vi "Untitled 6сщзн.vi"() -> ()   [LabVIEW 2021]
panel:
  in  "На улице":dbl
  in  "stop":bool
  out "XY Graph":cluster{i32[], dbl[]}[](graph)
  in  "Установка":dbl
  out "I":dbl
  in  "dt":dbl
  out "Даткчик":dbl
  out "IprevErr":dbl
  in  "kp":dbl
  in  "ki":dbl
  in  "kd":dbl
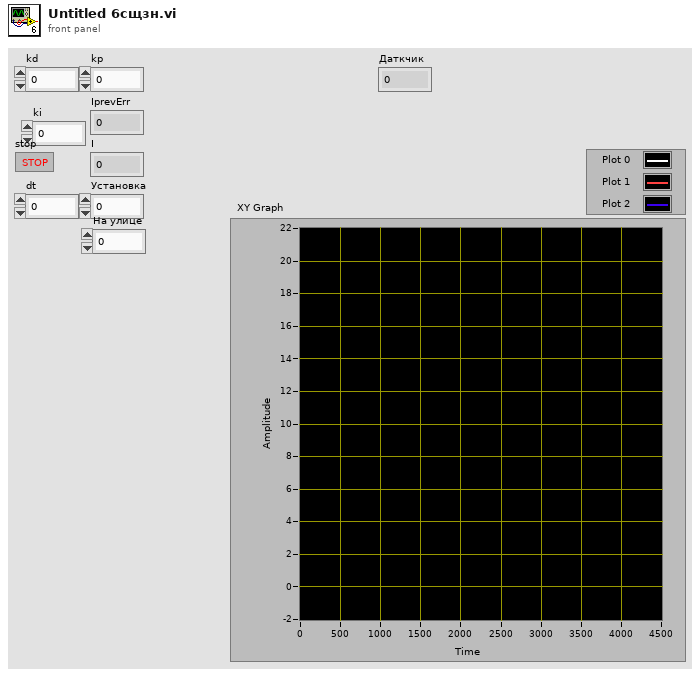
[diagram p1: front panel]
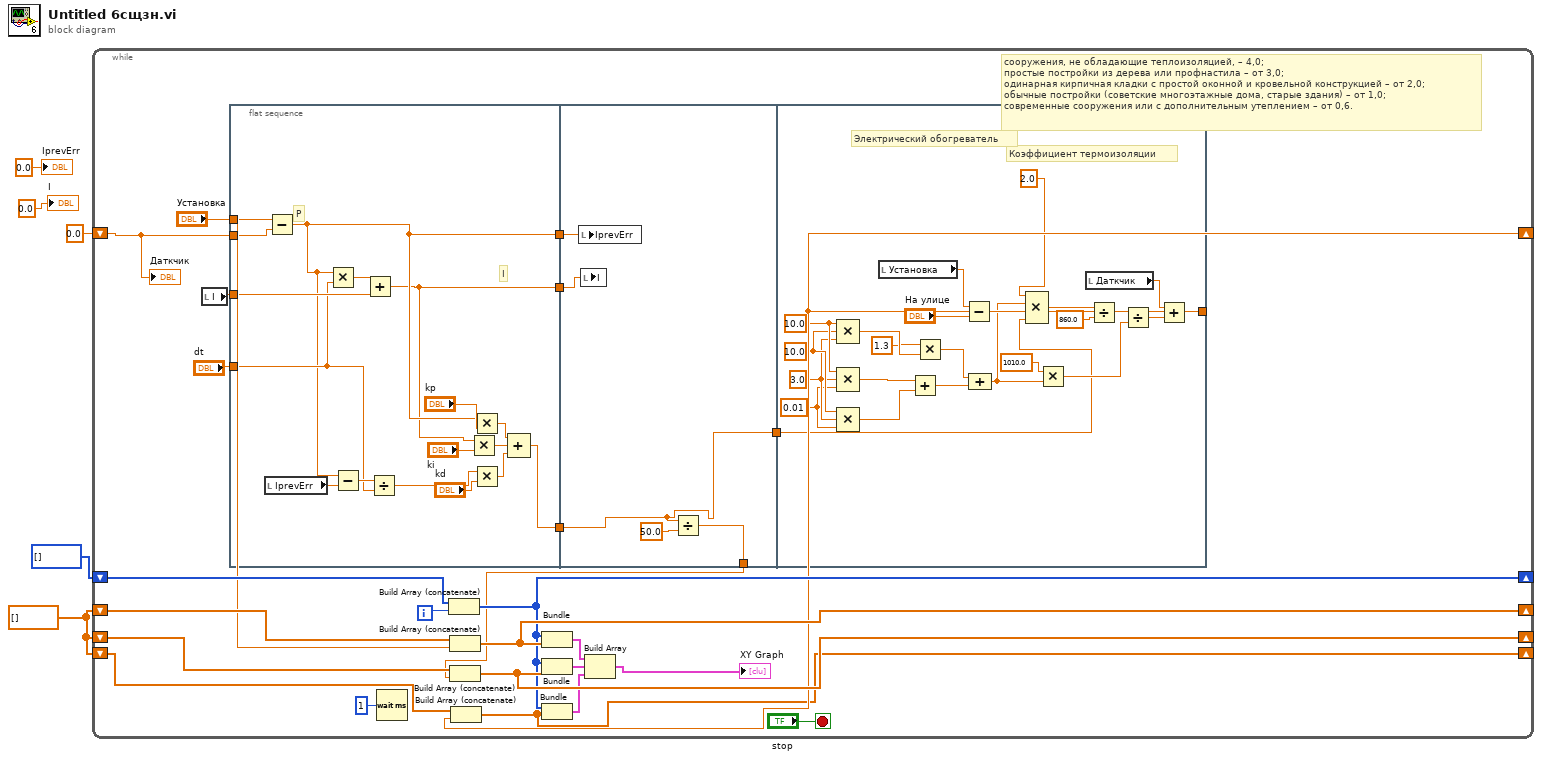
[diagram p0: block diagram]
diagram:
  w1 = dbl[] []
  n1 = while {
    shift-right: [w13] -> _
    shift-left: i32[] [] -> [w23]
    shift-right: [w17] -> _
    shift-left: w1 -> [w21]
    shift-right: [w9] -> _
    shift-left: 0.0 -> [w15]
    shift-right: [w18] -> _
    shift-left: w1 -> [w20]
    shift-right: [w8] -> _
    shift-left: w1 -> [w10]
    i -> [w24]
    stop <- "stop" stop-if-true
    # "сооружения, не обладающие теплоизоляцией, – 4,0;\nпростые постройки из дерева или профнастила – от 3,0;\nодинарная кирпичная кладки с простой оконной и кровельной конструкцией – от 2,0;\nобычные постройки (советские многоэтажные дома, старые здания) – от 1,0;\nсовременные сооружения или с дополнительным утеплением – от 0,6."
    n2 = local read "I"() -> (w29:dbl)
    n3 = flat-sequence {
      tunnel: "Установка" -> [w37]
      tunnel: w15 -> [w31]
      tunnel: w29 -> [w36]
      tunnel: "dt" -> [w35]
      tunnel: [w34] -> w27
      tunnel: [w33] -> w26
      tunnel: [w32] -> w25
      tunnel: w27 -> [w49]
      tunnel: w26 -> [w52]
      tunnel: w25 -> [w51]
      tunnel: [w49] -> w7
      tunnel: [w48] -> w6
      tunnel: [w75] -> w9
      tunnel: w7 -> [w54]
      frame #0 {
        # "I"
        # "P"
        n4 = local read "IprevErr"() -> (w39:dbl)
        n5 = Subtract(x=w37, y=w31) -> (x-y=w33:dbl)
        n6 = Multiply(x=w33, y=w35) -> (x*y=w38:dbl)
        n7 = Subtract(x=w33, y=w39) -> (x-y=w40:dbl)
        n8 = Add(x=w38, y=w36) -> (x+y=w32:dbl)
        n9 = Divide(x=w40, y=w35) -> (x/y=w44:dbl)
        n10 = Multiply(x=w32, y="ki") -> (x*y=w42:dbl)
        n11 = Multiply(x=w33, y="kp") -> (x*y=w41:dbl)
        n12 = Multiply(x=w44, y="kd") -> (x*y=w43:dbl)
        n13 = Compound Arithmetic op=ADD(w41, w42, w43) -> (w34:dbl)
      }
      frame #1 {
        n14 = local write "IprevErr"(w52) -> ()
        n15 = local write "I"(w51) -> ()
        n16 = Divide(x=w49, y=50.0) -> (x/y=w48:dbl)
      }
      frame #2 {
        w69 = 0.01 ("value")
        w71 = 10.0 ("value")
        w70 = 3.0 ("value")
        w72 = 10.0 ("value")
        # "Электрический обогреватель"
        # "Коэффициент термоизоляции"
        n17 = Compound Arithmetic op=MULTIPLY(w72, w71, w70) -> (w74:dbl)
        n18 = Compound Arithmetic op=MULTIPLY(w72, w70, w69) -> (w67:dbl)
        n19 = Compound Arithmetic op=MULTIPLY(w71, w70, w69) -> (w66:dbl)
        n20 = local read "Установка"() -> (w64:dbl)
        n21 = Add(x=w67, y=w66) -> (x+y=w65:dbl)
        n22 = Multiply(x=1.3 ("value"), y=w74) -> (x*y=w68:dbl)
        n23 = Subtract(x=w64, y="На улице") -> (x-y=w61:dbl)
        n24 = Compound Arithmetic op=unknown(w68, w65) -> (w57:dbl)
        n25 = Compound Arithmetic op=MULTIPLY(2.0 ("value"), w57, w61, w54) -> (w60:dbl)
        n26 = Multiply(x=1010.0, y=w57) -> (x*y=w56:dbl)
        n27 = local read "Даткчик"() -> (w76:dbl)
        n28 = Divide(x=w60, y=860.0) -> (x/y=w53:dbl)
        n29 = Divide(x=w53, y=w56) -> (x/y=w55:dbl)
        n30 = Add(x=w76, y=w55) -> (x+y=w75:dbl)
      }
    }
    n31 = Wait (ms)(milliseconds to wait=u32 1) -> ()  [unwired: 1 out]
    n32 = Build Array (concatenate)(w23, w24) -> (w13:i32[])
    n33 = Build Array (concatenate)(w21, "Установка") -> (w17:dbl[])
    n34 = Build Array (concatenate)(w20, w6) -> (w18:dbl[])
    n35 = Build Array (concatenate)(w10, w9) -> (w8:dbl[])
    n36 = Bundle(w13, w17) -> (w30:cluster{i32[], dbl[]})  [unwired: 1 in]
    n37 = Bundle(w13, w18) -> (w12:cluster{i32[], dbl[]})  [unwired: 1 in]
    n38 = Bundle(w13, w8) -> (w11:cluster{i32[], dbl[]})  [unwired: 1 in]
    n39 = Build Array(w30, w12, w11) -> (→"XY Graph":cluster{i32[], dbl[]}[])
    "Даткчик" <- w15
  }
  "IprevErr" <- 0.0 ("IprevErr")
  "I" <- 0.0 ("IprevErr")
